vi "Global Variables.vi"() -> ()   [LabVIEW 2014]
panel:
  in  "Middle Encoder":dbl
  in  "Right Encoder":dbl
  in  "Left Encoder":dbl
  in  "Gyro Heading":dbl
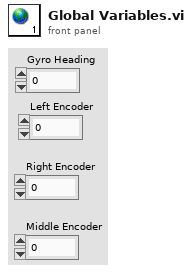
[diagram p1: front panel]
diagram:
